vi "New.vi"(7 "Parent":refnum<class "NonTerminal.lvclass">, 8 "Error In":errorcluster, 11 "Key":string) -> (0 "Error Out":errorcluster, 3 "Escaped Tag":refnum<class "EscapedTag.lvclass">)   [LabVIEW 2018, in "Toolkit.lvlib" / "Nodes.lvlib" / "EscapedTag.lvclass"]
uses:
  EscapedTag.lvclass
  NonTerminal/NonTerminal.lvclass
  D:/Users/cfield/Code/Field R&D Services/Mustache/trunk/src/Toolkit/Nodes/Abstract/Abstract.lvclass
  EscapedTag.lvclass/EscapedTag.ctl
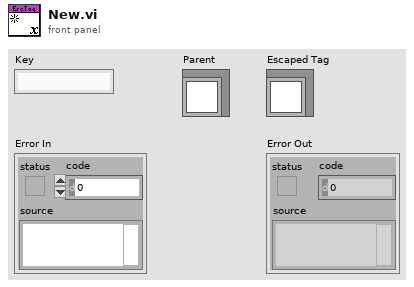
[diagram p1: front panel]
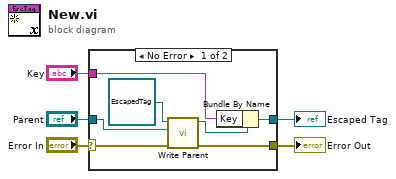
[diagram p0: block diagram]
diagram:
  n1 = case shown="No Error" "Error In" {
    selector: "Error In" -> [w8 w13]
    tunnel: [w7 w13] -> w5
    tunnel: "Key" -> [w11 _]
    tunnel: [w12 _] -> w1
    tunnel: "Parent" -> [w9 _]
    frame No Error {
      n2 = call-dynamic "Write Parent.vi"("Error In"=w8, "Parent"=w9, "Node In"=refnum<class "EscapedTag.lvclass"> refnum ("Toolkit.lvlib:Nodes.lvlib:EscapedTag.lvclass")) -> ("Error Out"=w7:errorcluster, "Node Out"=w6:refnum<class "EscapedTag.lvclass">)  [unwired: 7 in]
      n3 = Bundle By Name(cluster=w6, "Key"=w11) -> (w12:refnum<class "EscapedTag.lvclass">)
    }
    frame Error {
    }
  }
  "Error Out" <- w5
  "Escaped Tag" <- w1
